vi "Read dt.vi"(8 "error in (no error)":errorcluster, 11 "DCM-DSI-HW in":refnum<class "DCM-DSI.lvclass">) -> (0 "error out":errorcluster, 2 "dt CMD [s]":sgl, 3 "DCM-DSI-HW out":refnum<class "DCM-DSI.lvclass">)   [LabVIEW 2016, in "DCM-DSI.lvclass"]
uses:
  DCM-DSI.lvclass
  DCM-DSI.lvclass/DCM-DSI.ctl
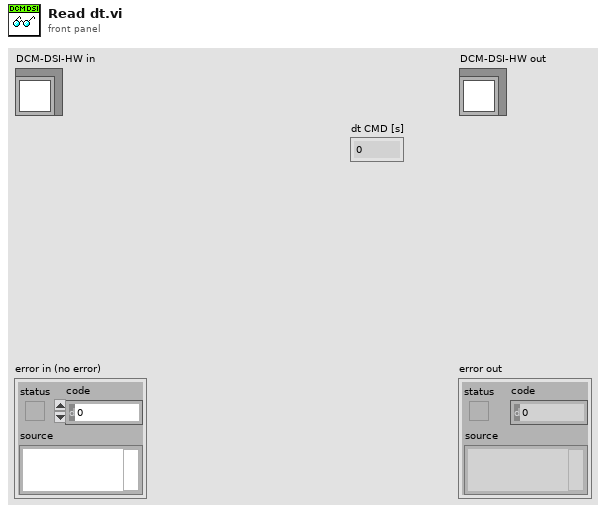
[diagram p1: front panel]
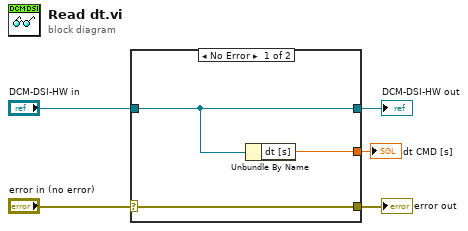
[diagram p0: block diagram]
diagram:
  n1 = case shown="No Error" "error in (no error)" {
    selector: "error in (no error)" -> [w8 w10]
    tunnel: [w8 w10] -> w4
    tunnel: [w7 w9] -> w2
    tunnel: "DCM-DSI-HW in" -> [w7 w9]
    tunnel: [w6 _] -> w1
    frame No Error {
      n2 = Unbundle By Name(w7) -> ("dt [s]"=w6:dbl)
    }
    frame Error {
    }
  }
  "error out" <- w4
  "DCM-DSI-HW out" <- w2
  "dt CMD [s]" <- w1
